vi "TestGetLocalizedPhrase.vi"(8 "error in (no error)":errorcluster) -> (0 "error out":errorcluster)   [LabVIEW 2017]
uses:
  <vilib>/addons/_JKI Toolkits/Caraya/classes/Test/Test.lvclass
  src/API/JKI Simple Localization.lvlib
  <vilib>/addons/_JKI Toolkits/Caraya/classes/Assert/Assert.lvclass
panel:
  # "See block diagram for unit tests of Get Localized Phrase.vi"
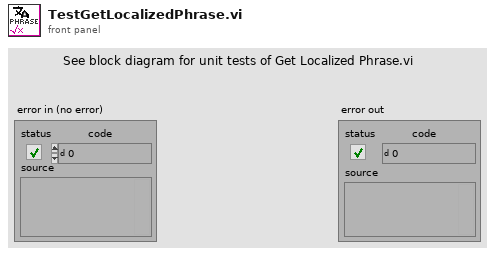
[diagram p1: front panel]
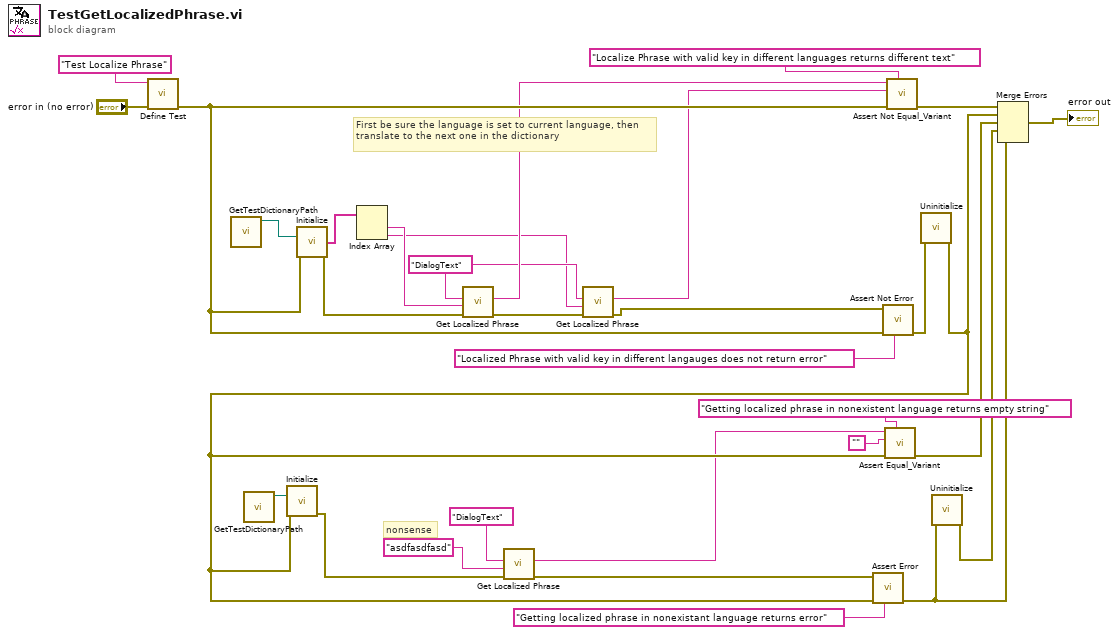
[diagram p0: block diagram]
diagram:
  w12 = "DialogText" ("Key")
  # "nonsense"
  # "First be sure the language is set to current language, then translate to the next one in the dictionary"
  n1 = call <vilib>:"Define Test.vi"("error in (no error)"="error in (no error)", "Label (VI Title)"="Test Localize Phrase") -> ("error out"=w22:errorcluster)  [unwired: 9 in]
  n2 = call "GetTestDictionaryPath.vi"() -> ("Test Dictionary Path"=w29:path)  [unwired: 11 in]
  n3 = call "GetTestDictionaryPath.vi"() -> ("Test Dictionary Path"=w24:path)  [unwired: 11 in]
  n4 = call "Initialize.vi"("Dictionary File Path"=w29, "error in"=w22) -> ("Languages"=w15:string[], "error out"=w16:errorcluster)  [unwired: 10 in, 2 out]
  n5 = Index Array(array=w15) -> (element #1=w14:string, element #2=w11:string)  [unwired: 2 in]
  n6 = call "Get Localized Phrase.vi"("error in"=w16, "Target Language (current lang)"=w14, "Key"=w12) -> ("error out"=w10:errorcluster, "Translated Phrase"=w13:string)  [unwired: 7 in]
  n7 = call "Get Localized Phrase.vi"("error in"=w10, "Target Language (current lang)"=w11, "Key"=w12) -> ("error out"=w8:errorcluster, "Translated Phrase"=w9:string)  [unwired: 7 in]
  n8 = call <vilib>:"Assert Not Error.vi"("Label"="Localized Phrase with valid key in different langauges does not return error", "error in (no error)"=w22, "Not Error?"=w8) -> ("error out"=w19:errorcluster)  [unwired: 8 in]
  n9 = call <vilib>:"Assert Not Equal_Variant.vi"("Label"="Localize Phrase with valid key in different languages returns different text", "error in (no error)"=w22, "Y"=w9, "X"=w13) -> ("error out"=w27:errorcluster)  [unwired: 7 in]
  n10 = call "Uninitialize.vi"("error in"=w19) -> ("error out"=w18:errorcluster)  [unwired: 10 in]
  n11 = call "Initialize.vi"("Dictionary File Path"=w24, "error in"=w18) -> ("error out"=w6:errorcluster)  [unwired: 10 in, 3 out]
  n12 = call "Get Localized Phrase.vi"("error in"=w6, "Target Language (current lang)"="asdfasdfasd", "Key"="DialogText") -> ("error out"=w5:errorcluster, "Translated Phrase"=w2:string)  [unwired: 7 in]
  n13 = call <vilib>:"Assert Error.vi"("Label"="Getting localized phrase in nonexistant language returns error", "error in (no error)"=w18, "Error?"=w5) -> ("error out"=w4:errorcluster)  [unwired: 8 in]
  n14 = call <vilib>:"Assert Equal_Variant.vi"("Label"="Getting localized phrase in nonexistent language returns empty string", "error in (no error)"=w18, "Y"="", "X"=w2) -> ("error out"=w20:errorcluster)  [unwired: 7 in]
  n15 = call "Uninitialize.vi"("error in"=w4) -> ("error out"=w17:errorcluster)  [unwired: 10 in]
  n16 = Merge Errors(w27, w18, w20, w17, w4) -> (→"error out":errorcluster)
